vi "RTD_close.vi"(7 "type":T2=enum."COMET Tx5xx (ethernet)" caption="Type", 8 "error in":errorcluster, 10 "thermo channel":T1={"type"=enum."COMET Tx5xx (ethernet)", "comment"="", "tag"="", "refresh"=5.0, "IP"="", "port"=502, "VISA"="", "last readout"=timestamp(0 s since 1904-01-01), "TCP ref"=refnum, "VISA sess"="", "idn"="", "press"=0.0, "RH"=0.0, "temp"=0.0, "pres cor"=[], "RH cor"=[], "temp cor"=[], "try left"=0, "failed"=FALSE, "RTD set"=[], "RTD inv"=[], "range"=0.0, "net mode"=enum."MODBUS", "try fail"=enum."Stop trying - return NaN", "timeout [s]"=0.0, "max retries"=0, "sim t [deg]"=0.0, "status"=0} {"status" items=["ok", "retry", "failed"]; "RTD inv" format="%.1f"; "RTD set" format="%.1f"; "temp cor" format="%.1f"; "RH cor" format="%.1f"; "pres cor" format="%.1f"; "refresh" min=0.1 max=1000.0 format="%.2f"}, 11 "VISA in":refnum<visa-resource-name>) -> (0 "error out":errorcluster)   [LabVIEW 2020]
uses:
  thermo_types.ctl
  thermo.ctl
  Thermometer Fail Action.ctl
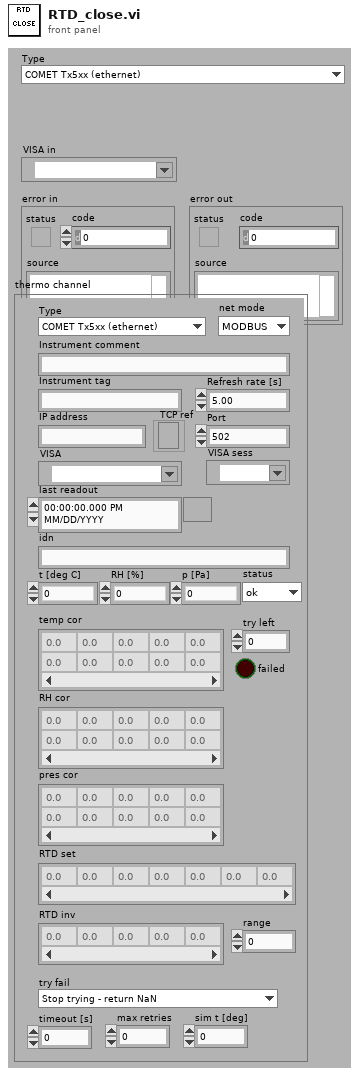
[diagram p1: front panel]
types:
  T1 = typedef "thermo.ctl" = cluster{"type":T2, "comment":string, "tag":string, "refresh":dbl, "IP":string, "port":u16, "VISA":refnum<visa-resource-name>, "last readout":timestamp, "TCP ref":refnum<k5>, "VISA sess":refnum<visa-resource-name>, "idn":string, "press":dbl, "RH":dbl, "temp":dbl, "pres cor":dbl[][], "RH cor":dbl[][], "temp cor":dbl[][], "try left":i32, "failed":bool, "RTD set":dbl[], "RTD inv":dbl[], "range":dbl, "net mode":enum16{"MODBUS", "HTTP"}, "try fail":T3, "timeout [s]":dbl, "max retries":i32, "sim t [deg]":dbl, "status":u16}
  T2 = typedef "thermo_types.ctl" = enum16{"Disabled", "Simulated", "COMET Tx5xx (ethernet)", "Keithley 2002 (GPIB) + RTD", "Agilent 344xx (GPIB) + RTD"}
  T3 = typedef "Thermometer Fail Action.ctl" = enum16{"Stop trying - keep last value", "Stop trying - return NaN", "Generate error - stop sweep"}
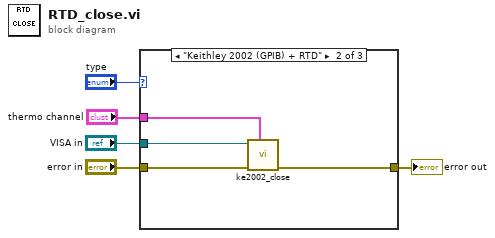
[diagram p0: block diagram]
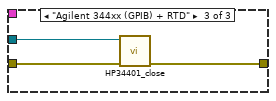
[diagram p3: hidden frame]
diagram:
  n1 = case shown="\"Keithley 2002 (GPIB) + RTD\"" "type" {
    tunnel: "error in" -> [w6 w10 w13]
    tunnel: [w6 w8 w12] -> w3
    tunnel: "VISA in" -> [_ w9 w11]
    tunnel: "thermo channel" -> [_ w7 _]
    frame Default {
    }
    frame "Keithley 2002 (GPIB) + RTD" {
      n2 = call "ke2002_close.vi"("thermo channel"=w7, "error in"=w10, "VISA in"=w9) -> ("error out"=w8:errorcluster)  [unwired: 8 in]
    }
    frame "Agilent 344xx (GPIB) + RTD" {
      n3 = call "HP34401_close.vi"("error in"=w13, "VISA in"=w11) -> ("error out"=w12:errorcluster)  [unwired: 9 in]
    }
  }
  "error out" <- w3
